vi "Complete_Controller_w_optics.vi"() -> ()   [LabVIEW 2014]
uses:
  <vilib>/LabVIEW Interface for Arduino/Type Defs/Arduino Resource.ctl
  <vilib>/LabVIEW Interface for Arduino/Type Defs/Board Type.ctl
  <vilib>/Instr/_visa.llb/VISA Configure Serial Port (Instr).vi
  <vilib>/Utility/file.llb/Write To Spreadsheet File (string).vi
  <vilib>/Utility/file.llb/Write To Spreadsheet File (DBL).vi
  <vilib>/Utility/file.llb/Read From Spreadsheet File (string).vi
  <vilib>/DAQmx/write.llb/DAQmx Write (Digital Bool 1Line 1Point).vi
  <vilib>/DAQmx/write.llb/DAQmx Write (Analog 1D DBL NChan 1Samp).vi
  <vilib>/DAQmx/read.llb/DAQmx Read (Analog 1D DBL NChan 1Samp).vi
  Environmental Chamber LabVIEW and Instruments/Drivers and Software/keithley_6430/Keithley 6430/Public/Data/Read (Single Point).vi
  Environmental Chamber LabVIEW and Instruments/Drivers and Software/LabVIEW 8.2 Drivers/keithley_24xx/Keithley 24XX/Public/Data/Read (Single Point).vi
  Environmental Chamber LabVIEW and Instruments/Drivers and Software/keithley_24xx/Keithley 24XX/Keithley 24XX.lvlib
  Environmental Chamber LabVIEW and Instruments/Drivers and Software/keithley_6430/Keithley 6430/Keithley 6430.lvlib
  <vilib>/LabVIEW Interface for Arduino/LabVIEW Interface for Arduino.lvlib
panel:
  in  "Integration Time (ms)":i32=80 caption="Inter scan delay ms"
  in  "Optical Smoothing Level":i32 min=0 max=4 step=1
  in  "Number of Scans to Average":i32=1 min=1 max=10000 step=1
  in  "Digitizer Clock Rate Setting":i32=3 min=1 max=3
  out "Critical Error":bool
  in  "Save spectra file path":path=path "C:/Users/User/Desktop/Chamber Data/perovskites/2015-08-04 spectra"
  in  "Aquire spectra":bool
  in  "Seconds between  spectra":dbl caption="Time Target (s)"
  out "Spectrum":cluster{"Wavelengths":dbl[], "buffer out":sgl[]}(graph)
  out "output param":i32
  out "Sequence time left (hrs)":dbl caption="min"
  out "Sequence Preview":cluster{dbl[], dbl[]}[](graph)
  out "Pressure Control 3":bool caption="Pressure Control"
  in  "valve % open":dbl=100.0 min=0.0 max=100.0 step=5.0
  in  "Vapor\nflow\n(sccm)":sgl(slide) min=0 max=100 step=1 scale=0.0..200.0
  out "Actual":dbl
  out "Boolean 3":bool
  out "Actual":dbl
  out "Boolean":bool
  in  "Gas\nflow\n(sccm)":sgl(slide) min=0 max=100 step=1 scale=0.0..200.0
  in  "Desired pressure":dbl min=0.0 max=760.0 step=5.0
  out "Valve position (%)":dbl
  in  "Pressure Control":enum32{"Set % open ", " Set pressure  (Torr)"}(radio)
  out "Pressure Control 2":bool caption="Pressure Control"
  out "Keithley 6430":bool
  out "J-Kem":bool caption="J-Kem Temp"
  out "J-Kem Temp (C)":cluster{dbl}(graph)
  out "Keithley 2420":bool caption="Keithley 2430"
  out "Pressure Control":bool
  out "SRS QCM":bool
  out "MHz":dbl format="%.6f"
  out "Ohm":dbl format="%.4e"
  out "Waveform Chart 7":cluster{dbl, "Resistance out":dbl}(graph)
  out "Chamber Pressure (Torr)":cluster{"f":dbl}(graph)
  in  "Start recording after":dbl caption="min"
  in  "Auto stop after":bool
  in  "hrs":dbl=1000.0 min=0.0
  out "Start Time":string
  out "Elapsed (min)":dbl caption="Elapsed Time (s)"
  in  "Delay between data points (s)":dbl caption="sec" min=0.0 max=30.0 format="%#_13g"
  in  "Turbo pump auto on":bool
  in  "stop":bool
  in  "Experiment Notes":string
  in  "Clear all charts":bool
  out "Save data file path":path
  out "Waveform Chart 2":cluster{"f":dbl, "f":dbl}(graph)
  out "Keithley 2420 (Ohm)":cluster{"Resistance":sgl}(graph)
  out "Keithley 6430 (Ohm)":cluster{"Measurement":dbl}(graph)
  in  "Tab Control":T1(tab)
  out "run sequence table":string[][](table) caption="Sequence to run"
  in  "Run Sequence":bool
  out "Current step":i32
  out "Step time remaining (min)":dbl caption="min" format="%#_1g"
  in  "Import sequence file":path
  in  "Use excel file\nfor sequence?":bool
  in  "Pressure Mode":T2(radio)
  in  "User-defined\nsequence":string[][](table) caption="Create sequence"
  in  "Partial pressure of solvent (%)":dbl=100.0 min=0.0 max=100.0 step=5.0
  out "Arduino":bool
  out "temp\n(C)":string
  out "gas\nsensor":string
  out "Arduino humidity (%)":cluster{dbl}(graph)
  out "QCM mass deposited (g)":cluster{dbl}(graph)
  in  "rapidox O2 Sensor":bool
  in  "setnag O2 Pump":bool
  in  "Baud Rate 2":i32(ring)=2 items=["2400", "4800", "9600", "19200", "38400", "57600", "115200"]
  in  "Com Port":i32(ring) items=["Com 1", "Com 2", "Com 3", "Com 4", "Com 5", "Com 6", "COM 7", "COM 8", "COM 9", "COM 10", "COM 11", "COM 12", "com 13", "COM 14"]
  in  "Com Port 2":i32(ring) items=["Com 1", "Com 2", "Com 3", "Com 4", "Com 5", "Com 6", "COM 7", "COM 8", "COM 9", "COM 10", "COM 11", "COM 12", "com 13", "COM 14"]
  out "Torr":dbl
  out "%":dbl
  out "atm":dbl
  out "Waveform Chart":cluster{dbl}(graph)
  out "O2 Concentration (PPM)":dbl
  out "Waveform Chart 6":cluster{dbl}(graph)
  # "Currently Unused"
  # "QCM"
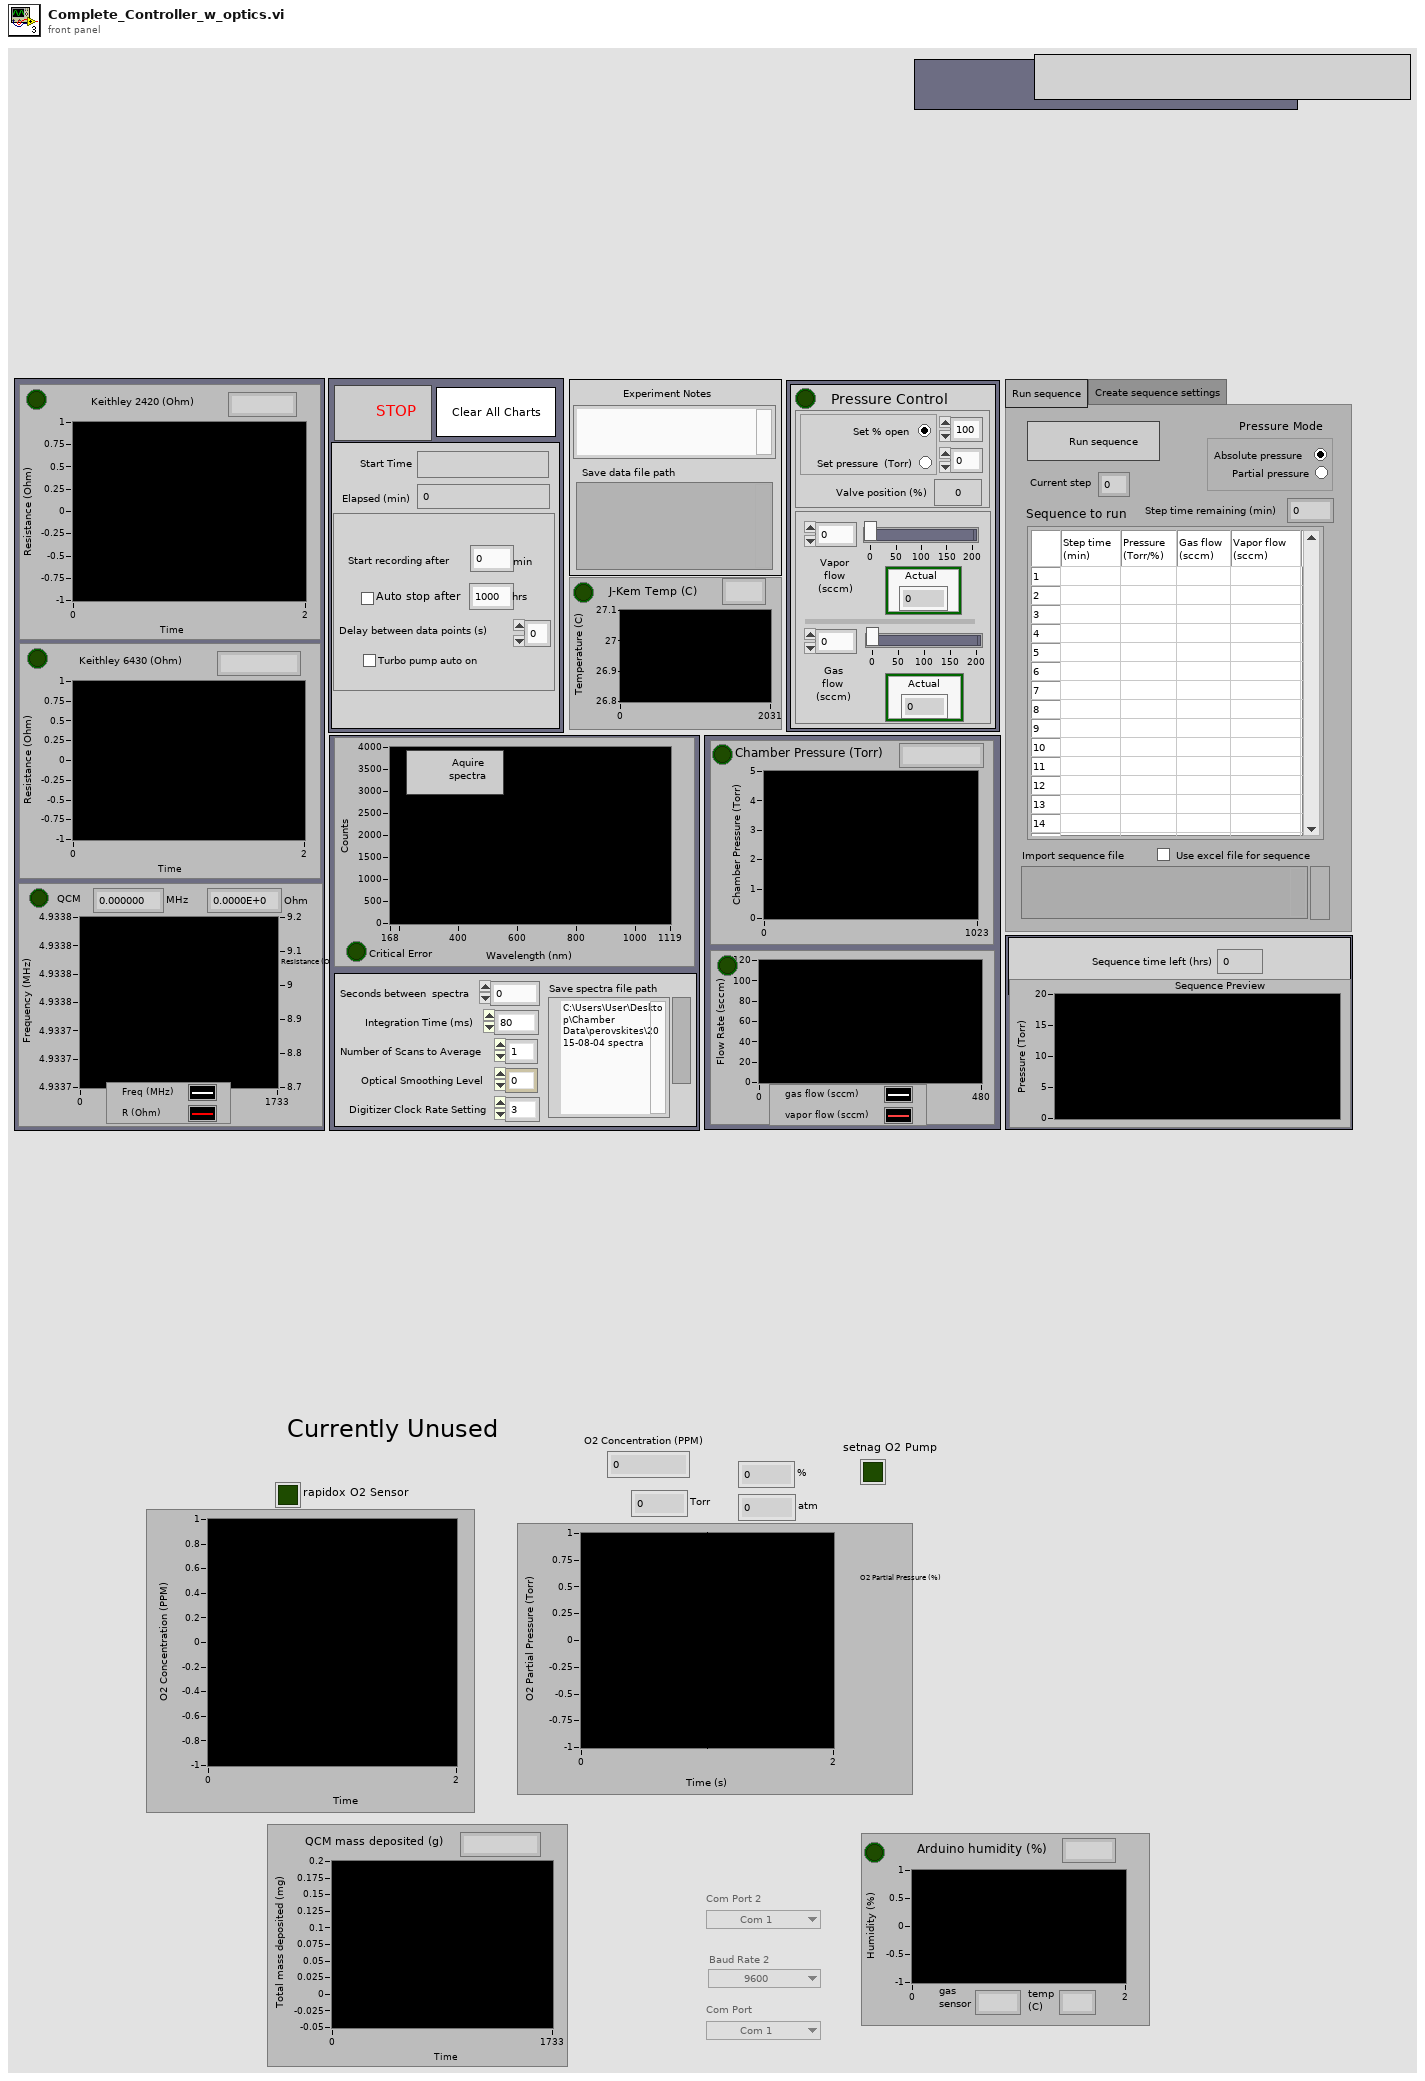
[diagram p1: front panel]
types:
  T1 = enum32{"Run sequence", "Create sequence settings"}
  T2 = enum32{"Absolute pressure ", " Partial pressure"}
  T3 = enum16{"open", "open or create", "create or replace", "create", "open (read only)"}
  T4 = enum16{"no parity", "odd parity", "even parity", "mark parity", "space parity"}
  T5 = cluster{bool, "VISA resource name":refnum<visa-resource-name>, "error out":errorcluster}
  T6 = cluster{bool, "VISA resource name out":refnum<visa-resource-name>, "error out":errorcluster}
  T7 = cluster{"task out":refnum<k21>, "error out":errorcluster, "task out":refnum<k21>, "error out":errorcluster, "task out":refnum<k21>, "error out":errorcluster, "VISA resource name":refnum<visa-resource-name>, "error out":errorcluster}
  T8 = cluster{"task out":refnum<k21>, "error out":errorcluster, "task out":refnum<k21>, "error out":errorcluster, "task out":refnum<k21>, "error out":errorcluster, "VISA resource name out":refnum<visa-resource-name>, "error out":errorcluster}
  T9 = cluster{"Coefficients":ext[], "Wavelengths":dbl[]}[]
  T10 = cluster{"Integration Time (ms)":i32, "Number of Scans to Average":i32, "Optical Smoothing Level":i32, "Digitizer Clock Rate Setting":i32, "Temp  Compensation ":bool}[]
  T11 = cluster{"Integration Time (ms)":i32, "Number of Scans to Average":i32, "Optical Smoothing Level":i32, "Digitizer Clock Rate Setting":i32, "Temp  Compensation ":bool}
  T12 = cluster{"Coefficients":ext[], "Wavelengths":dbl[]}
  T13 = cluster{bool, "VISA out":refnum<visa-resource-name>, "error out":errorcluster}
  T14 = cluster{"Boolean":bool, "VISA resource name out":refnum<visa-resource-name>, "error out":errorcluster}
  T15 = typedef "LabVIEW Interface for Arduino.lvlib/Arduino Resource.ctl" = cluster{"VISA resource":refnum<visa-resource-name>, "Board Type":T16, "Connection Type":enum8{"USB / Serial"}, "Bytes Per Packet (15)":u8}
  T16 = typedef "LabVIEW Interface for Arduino.lvlib/Board Type.ctl" = enum16{"Uno", "Dimuelanove w/Atmega 328", "Mega 2560"}
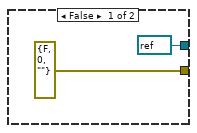
[diagram p3: hidden frame]
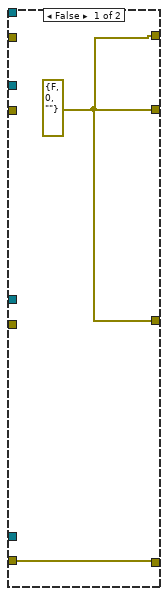
[diagram p4: hidden frame]
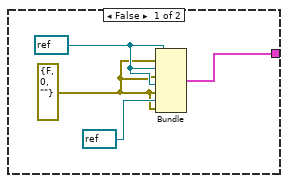
[diagram p5: hidden frame]
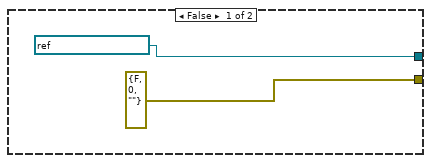
[diagram p7: hidden frame]
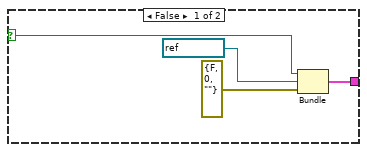
[diagram p8: hidden frame]
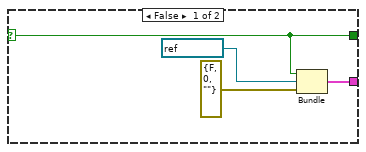
[diagram p10: hidden frame]
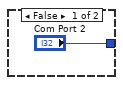
[diagram p11: hidden frame]
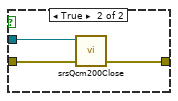
[diagram p12: hidden frame]
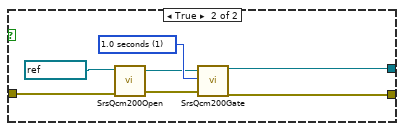
[diagram p13: hidden frame]
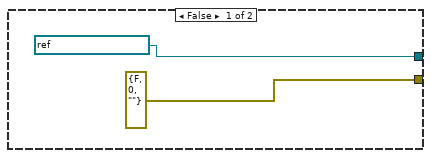
[diagram p15: hidden frame]
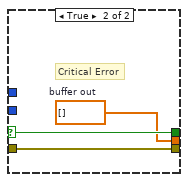
[diagram p17: hidden frame]
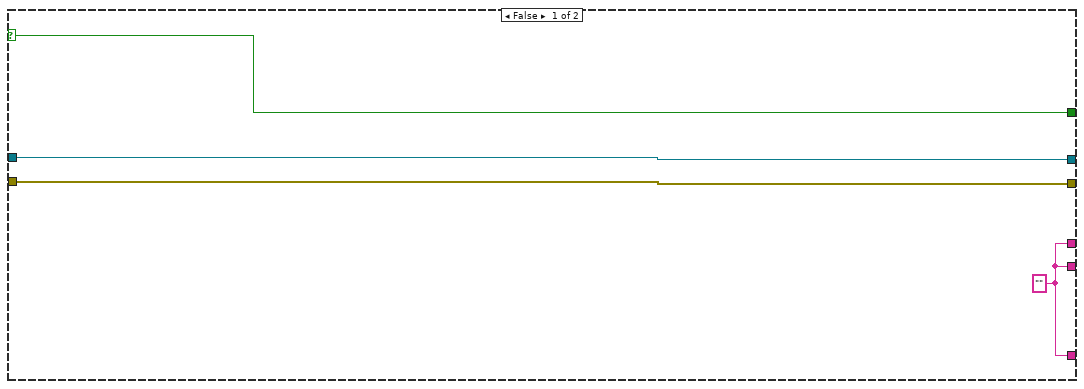
[diagram p18: hidden frame]
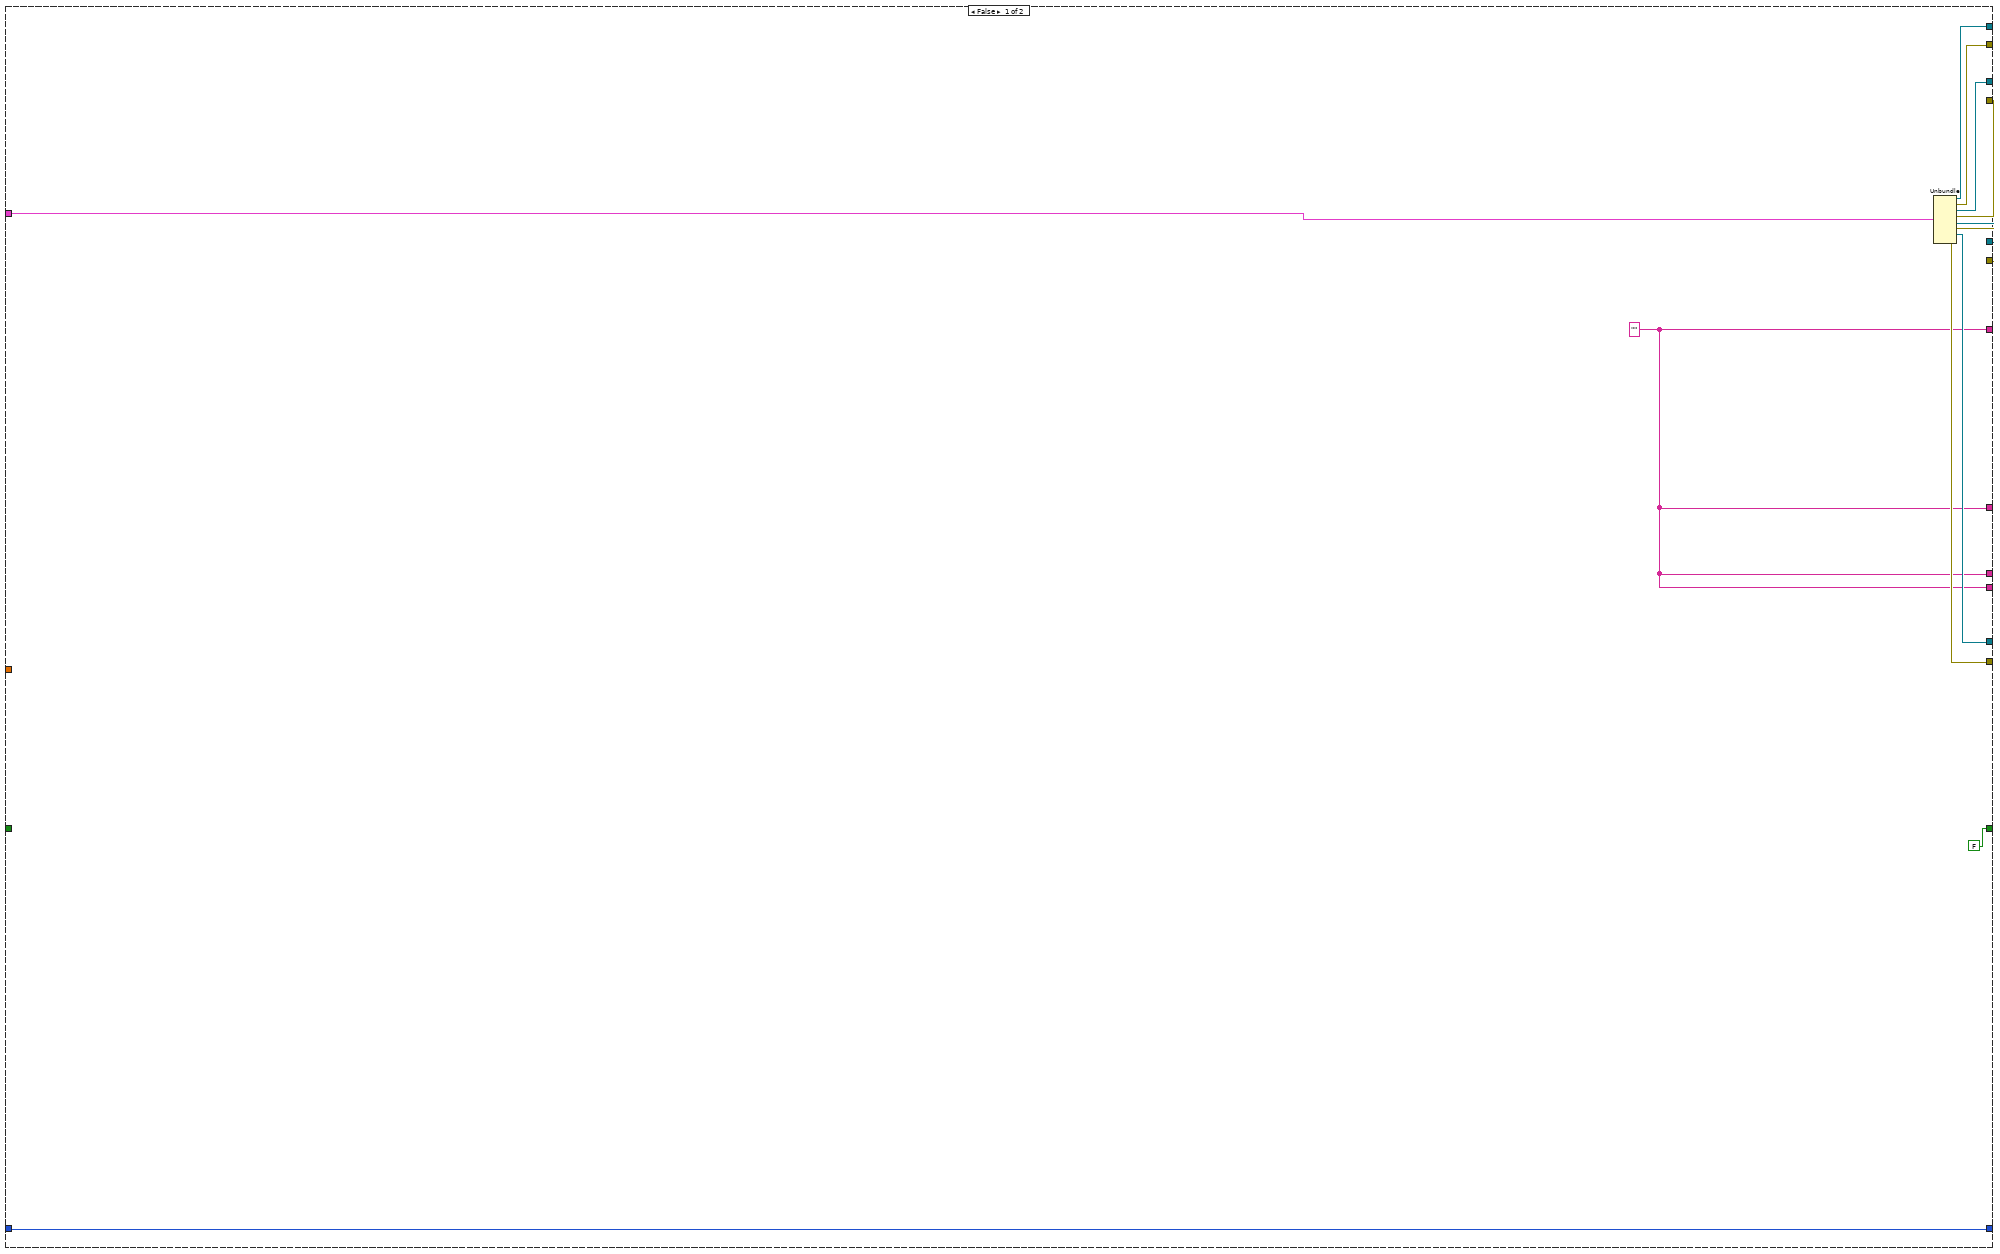
[diagram p19: hidden frame]
diagram:
  w29 = 0  # 1st step
  n1 = call "setup.vi"() -> ("Save file path 2"=w1:path, "begin recording"=w16:dbl, "error IO"=w4:errorcluster, "stop after"=w18:dbl, "Auto Stop 2"=w19:bool, "delay 5"=w17:dbl, "SRS QCM 2"=w15:bool, "Keithley 6431"=w11:bool, "Keithley 2421"=w14:bool, "J-KEM2"=w13:bool, "Arduino2"=w12:bool, "Pressure control 2"=w10:bool)  [unwired: 8 in]
  "SRS QCM" <- w15
  "Arduino" <- w12
  "Pressure Control" <- w10
  "Keithley 2420" <- w14
  "J-Kem" <- w13
  "Keithley 6430" <- w11
  "Pressure Control 2" <- w10
  "Pressure Control 3" <- w10
  n2 = local write "Auto stop after"(w19) -> ()
  n3 = local write "hrs"(w18) -> ()
  n4 = local write "Delay between data points (s)"(w17) -> ()
  n5 = local write "Start recording after"(w16) -> ()
  n6 = case shown="True" w14 {
    tunnel: [refnum<visa-resource-name> "GPIB1::24::INSTR" ("VISA resource name") w108] -> w96
    tunnel: [errorcluster {"status"=FALSE, "code"=0, "source"=""} ("error out") w103] -> w95
    frame False {
    }
    frame True {
      w110 = u16 0 items=["Voltage", "Current"] ("Source Mode  (0: Voltage)")
      w115 = u16 2 items=["Volts", "Current", "Resistance"] ("Function (0: Volts)")
      n7 = call "Initialize.vi"("VISA resource name"=refnum<visa-resource-name> "GPIB1::24::INSTR") -> ("error out"=w104:errorcluster, "VISA resource name out"=w107:refnum<visa-resource-name>)  [unwired: 9 in]
      n8 = call "Enable Remote Sensing.vi"("error in (no error)"=w104, "Enable Remote Sensing (T: Enable)"=FALSE ("4-wire?"), "VISA resource name"=w107) -> ("error out"=w105:errorcluster, "VISA resource name out"=w106:refnum<visa-resource-name>)  [unwired: 7 in]
      n9 = call "Configure Measurement.vi"("error in (no error)"=w105, "Function (0: Volts)"=w115, "VISA resource name"=w106) -> ("error out"=w114:errorcluster, "VISA resource name out"=w113:refnum<visa-resource-name>)  [unwired: 7 in]
      n10 = call "Configure Output.vi"("Source Mode  (0: Voltage)"=w110, "error in (no error)"=w114, "Output Level (0)"=0.1 ("Applied Voltage (V)"), "VISA resource name"=w113) -> ("error out"=w112:errorcluster, "VISA resource name out"=w111:refnum<visa-resource-name>)  [unwired: 6 in]
      n11 = call "Enable Output.vi"("error in (no error)"=w112, "VISA resource name"=w111) -> ("error out"=w103:errorcluster, "VISA resource name out"=w108:refnum<visa-resource-name>)  [unwired: 8 in]
    }
  }
  n12 = case shown="True" w11 {
    tunnel: [refnum<visa-resource-name> "GPIB0::29::INSTR" ("VISA resource name") w125] -> w53
    tunnel: [errorcluster {"status"=FALSE, "code"=0, "source"=""} ("error out") w126] -> w52
    frame False {
    }
    frame True {
      (unwired) 15000.0 ("Resistance Range [Ohms]")
      w121 = u16 0 items=["On", "Off", "Once"] ("Autozero  (0: On)")
      w129 = TRUE  # Output (F:Off)
      n13 = call "Initialize.vi"("VISA resource name"=refnum<visa-resource-name> "GPIB0::29::INSTR") -> ("error out"=w122:errorcluster, "VISA resource name out"=w123:refnum<visa-resource-name>)  [unwired: 4 in, 5 out]
      n14 = call "Configure Autozero.vi"("error in (no error)"=w122, "Autozero  (0: On)"=w121, "VISA resource name"=w123) -> ("error out"=w119:errorcluster, "VISA resource name out"=w120:refnum<visa-resource-name>)  [unwired: 7 in]
      n15 = call "Configure MeasureOhms.vi"("error in (no error)"=w119, "Auto Range (T:Enable)"=TRUE, "VISA resource name"=w120) -> ("error out"=w130:errorcluster, "VISA resource name out"=w128:refnum<visa-resource-name>)  [unwired: 3 in, 4 out]
      n16 = call "Enable Output.vi"("error in (no error)"=w130, "Enable Output (F:Off)"=w129, "VISA resource name"=w128) -> ("error out"=w126:errorcluster, "VISA resource name out"=w125:refnum<visa-resource-name>)  [unwired: 7 out]
    }
  }
  n17 = property on="Turbo pump auto on" class="Bool (strict)"(error in=w4, "Value"=TRUE ("Turbo\npump")) -> (error out=w3:errorcluster)  [unwired: 1 in, 1 out]
  n18 = case shown="True" "setnag O2 Pump" {
    tunnel: ["Com Port 2" w132] -> w92
    frame False {
    }
    frame True {
      n19 = flat-sequence {
        tunnel: ["Com Port"] -> w135
        tunnel: [w137] -> w134
        tunnel: ["Com Port"] -> w133
        tunnel: w135 -> [w143]
        tunnel: w134 -> [w142]
        tunnel: w133 -> [w144]
        tunnel: [w144] -> w132
        frame #0 {
          n20 = property on="Baud Rate 2" class="Ring (strict)"() -> ("Strings []"=w139:string[])  [unwired: 2 in, 2 out]
          n21 = Index Array(array=w139, index="Baud Rate 2") -> (element=w140:string)
          n22 = Decimal String To Number(string=w140) -> (number=w138:i32)  [unwired: 2 in, 1 out]
          n23 = To Unsigned Long Integer(number=w138) -> (unsigned 32bit integer=w137:u32)
        }
        frame #1 {
          n24 = call <vilib>:"Serial Port Init.vi"("parity"=T4."no parity", "buffer size"=u16 65535, "stop bits"=enum16{"1 bit", "1.5 bits", "2 bits"}."1 bit", "data bits"=u16 8, "baud rate"=w142, "port number"=w143) -> ()  [unwired: 1 in, 1 out]
        }
      }
    }
  }
  n25 = property on="Run Sequence" class="Bool (strict)"(error in=w3, "Value"=FALSE ("Run Sequence")) -> (error out=w8:errorcluster)  [unwired: 1 in, 1 out]
  n26 = case shown="True" "rapidox O2 Sensor" {
    selector: "rapidox O2 Sensor" -> [w149 w154]
    tunnel: [w150 w155] -> w63
    frame False {
      n27 = Bundle(w149, "VISA resource name"=refnum<visa-resource-name> "COM7", "error out"=errorcluster {"status"=FALSE, "code"=0, "source"=""}) -> (w150:T5)  [unwired: 1 in]
    }
    frame True {
      n28 = call-poly "VISA Configure Serial Port"("VISA resource name"=refnum<visa-resource-name> "COM7") -> ("VISA resource name out"=w156:refnum<visa-resource-name>, "error out"=w153:errorcluster)  [unwired: 13 in]
      n29 = Bundle(w154, "VISA resource name out"=w156, "error out"=w153) -> (w155:T6)  [unwired: 1 in]
    }
  }
  n30 = case shown="False" w15 {
    tunnel: [refnum<visa-resource-name> "COM6" ("VISA in") w162] -> w94
    tunnel: [w158 w161] -> w93
    tunnel: w8 -> [w158 w160]
    frame False {
    }
    frame True {
      w166 = u16 1 items=["0.1 seconds", "1.0 seconds", "10.0 seconds"] ("Gate in")
      n31 = call "SrsQcm200Open.vi"("error in"=w160, "VISA in"=refnum<visa-resource-name> "COM6") -> ("error out"=w163:errorcluster, "VISA out"=w164:refnum<visa-resource-name>)  [unwired: 3 in]
      n32 = call "SrsQcm200Gate.vi"("VISA in"=w164, "Gate in"=w166, "error in (no error)"=w163) -> ("VISA out"=w162:refnum<visa-resource-name>, "error out"=w161:errorcluster)  [unwired: 14 in, 1 out]
    }
  }
  n33 = case shown="True" w10 {
    tunnel: [w167 w174] -> w34
    frame False {
      w169 = refnum<k21> refnum ("task out")
      w168 = errorcluster {"status"=FALSE, "code"=0, "source"=""} ("error out")
      n34 = Bundle("task out"=w169, "error out"=w168, "task out"=w169, "error out"=w168, "task out"=w169, "error out"=w168, "VISA resource name"=refnum<visa-resource-name> refnum, "error out"=w168) -> (w167:T7)  [unwired: 1 in]
    }
    frame True {
      # "Turbo Pump Control"
      # "DAQ Gas/Vapor Flow Readings"
      # "DAQ Pressure Readings"
      # "Butterfly Valve"
      n35 = call-poly "VISA Configure Serial Port"("VISA resource name"=refnum<visa-resource-name> "COM5") -> ("VISA resource name out"=w175:refnum<visa-resource-name>, "error out"=w171:errorcluster)  [unwired: 13 in]
      n36 = call <vilib>:"DAQmx Start Task.vi"("task/channels in"=refnum<k21> "AllDaqReadings") -> ("task out"=w177:refnum<k21>, "error out"=w176:errorcluster)  [unwired: 13 in]
      n37 = call <vilib>:"DAQmx Start Task.vi"("task/channels in"=refnum<k21> "TurboON") -> ("task out"=w181:refnum<k21>, "error out"=w180:errorcluster)  [unwired: 13 in]
      n38 = call <vilib>:"DAQmx Start Task.vi"("task/channels in"=refnum<k21> "Setflow") -> ("task out"=w179:refnum<k21>, "error out"=w178:errorcluster)  [unwired: 13 in]
      n39 = property on="Run Sequence" class="Bool (strict)"(error in=w171, "Value"=FALSE ("Run Sequence")) -> (error out=w173:errorcluster)  [unwired: 1 in, 1 out]
      n40 = Bundle("task out"=w181, "error out"=w180, "task out"=w179, "error out"=w178, "task out"=w177, "error out"=w176, "VISA resource name out"=w175, "error out"=w173) -> (w174:T8)  [unwired: 1 in]
    }
  }
  n41 = case shown="True" w13 {
    selector: w13 -> [w186 w191]
    tunnel: [w187 w192] -> w81
    tunnel: [w186 w191] -> w75
    frame False {
      n42 = Bundle(w186, "VISA resource name"=refnum<visa-resource-name> "COM3", "error out"=errorcluster {"status"=FALSE, "code"=0, "source"=""}) -> (w187:T5)  [unwired: 1 in]
    }
    frame True {
      n43 = call-poly "VISA Configure Serial Port"("VISA resource name"=refnum<visa-resource-name> "COM3") -> ("VISA resource name out"=w193:refnum<visa-resource-name>, "error out"=w190:errorcluster)  [unwired: 13 in]
      n44 = Bundle(w191, "VISA resource name out"=w193, "error out"=w190) -> (w192:T6)  [unwired: 1 in]
    }
  }
  n45 = Get Date/Time In Seconds() -> (seconds since 1Jan1904=w99:timestamp)
  n46 = case "Arduino" shown="True" w12 {
    tunnel: [refnum<visa-resource-name> refnum ("VISA resource name out") w200] -> w28
    tunnel: [errorcluster {"status"=FALSE, "code"=0, "source"=""} ("error out") w197] -> w27
    frame False {
    }
    frame True {
      n47 = call <vilib>:"Init.vi"() -> ()  [unwired: 18 in, 2 out]
      n48 = call-poly "VISA Configure Serial Port"("VISA resource name"=refnum<visa-resource-name> "COM12", "baud rate (9600)"=u32 9600) -> ("VISA resource name out"=w200:refnum<visa-resource-name>, "error out"=w197:errorcluster)  [unwired: 12 in]
    }
  }
  n49 = Format Date/Time String(seconds (now)=w99) -> (date/time string=→"Start Time":string)  [unwired: 2 in]
  n50 = call "OpenCreateReplace File.vi"("function (open:0)"=T3."create or replace", "file path"=w1) -> ("new file path"=w20:path)  [unwired: 6 in, 3 out]
  "Save data file path" <- w20
  n51 = while {
    shift-right: [w296] -> _
    shift-left: _ -> [w295]
    tunnel: [w225] -> w97 mode=indexing if=w224
    tunnel: w14 -> [w264]
    tunnel: w96 -> [w293]
    tunnel: w95 -> [w292]
    tunnel: w94 -> [w291]
    tunnel: w93 -> [w290]
    tunnel: w15 -> [w288]
    tunnel: "setnag O2 Pump" -> [w281]
    tunnel: w92 -> [w287]
    tunnel: [w283] -> w89
    tunnel: [w282] -> w85
    tunnel: w81 -> [w280]
    tunnel: [w279] -> w80
    tunnel: w75 -> [w277]
    tunnel: w63 -> [w273]
    tunnel: [w268] -> w61
    tunnel: [w263] -> w60
    tunnel: w20 -> [w263]
    shift-right: [w246] -> _
    shift-left: _ -> [w248]
    tunnel: w53 -> [w260]
    tunnel: w52 -> [w259]
    tunnel: [w258] -> w51
    tunnel: w11 -> [w257]
    tunnel: w10 -> [w238]
    tunnel: [w254] -> w47
    tunnel: [w253] -> w44
    tunnel: [w252] -> w46
    tunnel: [w251] -> w45
    tunnel: [w238] -> w43
    tunnel: [w250] -> w38
    tunnel: w34 -> [w242]
    tunnel: [w241] -> w32
    tunnel: [w240] -> w31
    tunnel: [w239] -> w30
    shift-right: [w237] -> _
    shift-left: w29 -> [w236]
    tunnel: w12 -> [w221]
    tunnel: w28 -> [w231]
    tunnel: w27 -> [w230]
    tunnel: [w229] -> w26
    tunnel: [w228] -> w25
    tunnel: [w227] -> w24
    shift-right: [w212] -> _
    shift-left: TRUE -> [w213]
    i -> [w210]
    stop <- w276 stop-if-true
    n52 = call "Elapsed Time"() -> ("Present (s)"=w235:dbl, "Elapsed Time (s)"=w275:dbl)  [unwired: 12 in, 6 out]
    n53 = call "Elapsed Time5"("Time Target (s)"="Seconds between  spectra", "Auto Reset"=TRUE) -> ("Time has Elapsed"=w204:bool)  [unwired: 10 in, 7 out]
    n54 = Divide(x=w275, y=60.0) -> (x/y=w215:dbl)
    "Elapsed (min)" <- w215
    n55 = And(x=w204, y="Aquire spectra") -> (x .and. y?=w202:bool)
    n56 = Greater Or Equal?(x=w215, y="Start recording after") -> (x >= y?=w224:bool)
    n57 = Multiply(x="hrs", y=60.0) -> (x*y=w207:dbl)
    n58 = case "Vacuum / Pressure / Sequence" shown="True" w238 {
      tunnel: [w395 w503] -> w253
      tunnel: [w396 w502] -> w251
      tunnel: [w398 w483] -> w254
      tunnel: [w397 w484] -> w252
      tunnel: [w396 w474] -> w250
      tunnel: [w391 w464] -> w245
      tunnel: [w391 w463] -> w244
      tunnel: [w391 w461] -> w243
      tunnel: w242 -> [w401 w459]
      tunnel: [w400 w450] -> w241
      tunnel: [w399 w449] -> w240
      tunnel: [w394 w448] -> w239
      tunnel: w236 -> [w393 w433]
      tunnel: [w393 w445] -> w237
      tunnel: w235 -> [_ w444]
      tunnel: w213 -> [_ w424]
      tunnel: [FALSE ("new element/subarray") w419] -> w212
      tunnel: [w391 w418] -> w211
      frame False {
        w391 = ""
        n59 = Unbundle(w401) -> ("task out"=w400:refnum<k21>, "error out"=w399:errorcluster, "task out"=w398:refnum<k21>, "error out"=w397:errorcluster, "task out"=w395:refnum<k21>, "error out"=w396:errorcluster, "VISA resource name out"=w394:refnum<visa-resource-name>)  [unwired: 1 out]
      }
      frame True {
        # "system info"
        # "DAQ Pressure, Gas/Vapor Flows, & Butterfly Valve Control"
        n60 = case shown="True" "Use excel file\nfor sequence?" {
          tunnel: ["User-defined\nsequence" w510] -> w410
          frame False {
          }
          frame True {
            n61 = call-poly <vilib>:"Read From Spreadsheet File.vi"("file path (dialog if empty)"="Import sequence file") -> ("all rows"=w512:string[][])  [unwired: 6 in, 4 out]
            n62 = for {
              tunnel: w512 -> [w514] mode=indexing
              tunnel: [w513] -> w510 mode=indexing
              n63 = for {
                tunnel: w514 -> [w516] mode=indexing
                tunnel: [w515] -> w513 mode=indexing
                n64 = Format Into String(w516) -> (resulting string=w515:string)  [unwired: 3 in, 1 out]
              }
            }
          }
        }
        "run sequence table" <- w410
        n65 = case shown="\" Partial pressure\"" "Pressure Mode" {
          tunnel: [w505 w507] -> w402
          tunnel: "Desired pressure" -> [w505 w506]
          frame "Absolute pressure ", Default {
          }
          frame " Partial pressure" {
            n66 = Divide(x=w506, y="Partial pressure of solvent (%)") -> (x/y=w507:dbl)
          }
        }
        n67 = Unbundle(w459) -> ("task out"=w452:refnum<k21>, "error out"=w451:errorcluster, "task out"=w453:refnum<k21>, "error out"=w454:errorcluster, "task out"=w455:refnum<k21>, "error out"=w456:errorcluster, "VISA resource name out"=w457:refnum<visa-resource-name>, "error out"=w458:errorcluster)
        n68 = Wait (ms)(milliseconds to wait=u32 1000) -> ()  [unwired: 1 out]
        n69 = Fract/Exp String To Number(string=w410) -> (number=w423:dbl[][])  [unwired: 3 in, 1 out]
        n70 = call "plot_usr_seq.vi"("User-defined sequence"=w410) -> ("Sequence Preview"=→"Sequence Preview":cluster{dbl[], dbl[]}[])
        n71 = Index Array(array=w423, index (col)=0 ("disabled index (col)")) -> (element=w437:dbl[])  [unwired: 1 in]
        n72 = Index Array "time"(array=w423, index (row)=0 ("disabled index (col)")) -> (element=w422:dbl[])  [unwired: 1 in]
        n73 = Add Array Elements(numeric array=w437) -> (sum=w428:dbl)
        n74 = Array Size(array=w422) -> ()  [unwired: 1 out]
        n75 = call-poly <vilib>:"DAQmx Read.vi"("task/channels in"=w455, "error in"=w456) -> ("task out"=w503:refnum<k21>, "data"=w494:dbl[], "error out"=w502:errorcluster)  [unwired: 11 in]
        n76 = And(x="Run Sequence", y=w424) -> (x .and. y?=w425:bool)
        n77 = case "Sequence" shown="True" w425 {
          tunnel: w444 -> [_ w553]
          tunnel: [w539 w554] -> w445
          tunnel: w433 -> [w539 w541]
          tunnel: "Vapor\nflow\n(sccm)" -> [w538 _]
          tunnel: "Gas\nflow\n(sccm)" -> [w537 _]
          tunnel: [w538 w562] -> w441
          tunnel: [w537 w561] -> w440
          tunnel: [w536 w560] -> w429
          tunnel: w402 -> [w536 _]
          tunnel: w423 -> [_ w547]
          tunnel: "Pressure Control" -> [w535 _]
          tunnel: [w535 enum32{"Open Mode", "Pressure Mode"}."Pressure Mode" ("Pressure Control")] -> w434
          tunnel: [0.0 w550] -> w427
          frame False {
          }
          frame True {
            # "User Sequence"
            n78 = Array Size(array=w547) -> (size(s)=w570:i32[])
            n79 = Index Array "gas flow"(array=w547, index (row)=w541, index (col)=2 ("disabled index (col)")) -> (element=w561:dbl)
            n80 = Index Array "Pressure"(array=w547, index (row)=w541, index (col)=1 ("disabled index (col)")) -> (element=w560:dbl)
            n81 = Index Array "vapor flow"(array=w547, index (row)=w541, index (col)=3 ("disabled index (col)")) -> (element=w562:dbl)
            n82 = Index Array "array length"(array=w570) -> (element=w548:i32)  [unwired: 1 in]
            n83 = Index Array "time"(array=w547, index (row)=w541, index (col)=0) -> (element=w559:dbl)
            n84 = Greater Or Equal?(x=w548, y=w541) -> (x >= y?=w567:bool)
            n85 = Multiply(x=w559, y=60.0) -> (x*y=w546:dbl)
            n86 = call "Elapsed Time3"("Time Target (s)"=w546, "Auto Reset"=TRUE, "Set Start Time (s)"=w553) -> ("Elapsed Time (s)"=w545:dbl, "Time has Elapsed"=w566:bool)  [unwired: 9 in, 6 out]
            n87 = Increment(x=w541) -> (x+1=→"Current step":i32)
            n88 = Subtract(x=w546, y=w545) -> (x-y=w542:dbl)
            n89 = And(x=w566, y=w567) -> (x .and. y?=w556:bool)
            n90 = call "Elapsed Time4"("Reset"=FALSE, "Set Start Time (s)"=w553) -> ("Elapsed Time (s)"=w551:dbl)  [unwired: 10 in, 7 out]
            n91 = Increment(x=w541) -> (x+1=w555:i32)
            n92 = Divide(x=w542, y=60.0) -> (x/y=→"Step time remaining (min)":dbl)
            n93 = Select(t=w555, s=w556, f=w541) -> (s? t:f=w554:i32)
            n94 = Divide(x=w551, y=60.0) -> (x/y=w550:dbl)
          }
        }
        n95 = Index Array "vapor flow"(array=w494, index=4) -> (element=w490:dbl)
        n96 = Index Array "vacuum presure"(array=w494, index=0) -> ()  [unwired: 1 out]
        n97 = Index Array "high pressure"(array=w494, index=1) -> (element=w497:dbl)
        n98 = Index Array "low pressure"(array=w494, index=2) -> (element=w468:dbl)
        n99 = Index Array "gas flow"(array=w494, index=3) -> (element=w492:dbl)
        n100 = Greater Or Equal To 0?(x=w468) -> (x >= 0?=w469:bool)
        n101 = Multiply(x=40.0, y=w490) -> (x*y=w481:dbl)
        n102 = Multiply(x=40.0, y=w492) -> (x*y=w478:dbl)
        n103 = Greater Or Equal?(x=w478, y=1.0) -> (x >= y?=w477:bool)
        n104 = Select(t=w468, s=w469, f=0.0) -> (s? t:f=w467:dbl)
        n105 = Greater Or Equal?(x=w481, y=1.0) -> (x >= y?=w480:bool)
        n106 = Multiply(x=100.0, y=w497) -> (x*y=w485:dbl)
        n107 = Select(t=w478, s=w477, f=0.0) -> (s? t:f=w412:dbl)
        "Actual" <- w412
        n108 = Select(t=w481, s=w480, f=0.0) -> (s? t:f=w411:dbl)
        "Actual" <- w411
        n109 = Greater?(x=w467, y=10.0) -> (0:w473:bool)
        n110 = Greater Or Equal To 0?(x=w485) -> (x >= 0?=w487:bool)
        n111 = Select(t=w485, s=w487, f=0.0) -> (s? t:f=w472:dbl)
        n112 = Bundle("f"=w412, "f"=w411) -> (→"Waveform Chart 2":cluster{"f":dbl, "f":dbl})  [unwired: 1 in]
        n113 = Greater Than 0?(x=w412) -> (x > 0?=→"Boolean 3":bool)
        n114 = Select(t=w472, s=w473, f=w467) -> (s? t:f=w414:dbl)
        n115 = Greater Than 0?(x=w411) -> (x > 0?=→"Boolean":bool)
        n116 = Greater?(x=0.05, y=w414) -> (0:w438:bool)
        n117 = Bundle("f"=w414) -> (→"Chamber Pressure (Torr)":cluster{"f":dbl})  [unwired: 1 in]
        n118 = And(x=w438, y="Turbo pump auto on") -> (x .and. y?=w446:bool)
        n119 = Number To Engineering String(4:w412) -> (0:w463:string)  [unwired: 3 in]
        n120 = Number To Engineering String(4:w414) -> (0:w464:string)  [unwired: 3 in]
        n121 = Number To Engineering String(4:w411) -> (0:w461:string)  [unwired: 3 in]
        n122 = Build Array(w441, w440) -> (w439:dbl[])
        n123 = Subtract(x=w428, y=w427) -> (x-y=w407:dbl)
        n124 = Equal To 0?(x=w412) -> (x = 0?=w416:bool)
        n125 = Equal To 0?(x=w411) -> (x = 0?=w417:bool)
        n126 = Divide(x=w407, y=60.0) -> (x/y=→"Sequence time left (hrs)":dbl)
        n127 = And(x=w416, y=w417) -> (x .and. y?=w415:bool)
        n128 = case shown="False" w415 {
          tunnel: w414 -> [w518 w528]
          tunnel: [w517 w527] -> w413
          tunnel: w412 -> [w526 _]
          tunnel: w411 -> [w524 _]
          frame False {
            # "Calculate humidity when gas/vapor are flowing"
            n129 = Add(x=w526, y=w524) -> (x+y=w525:dbl)
            n130 = Divide(x=w524, y=w525) -> (x/y=w519:dbl)
            n131 = Multiply(x=w518, y=w519) -> (x*y=w520:dbl)
            n132 = Divide(x=w520, y=23.8) -> (x/y=w522:dbl)
            n133 = Multiply(x=w522, y=100.0) -> (x*y=w517:dbl)
          }
          frame True {
            # "calculate humidity when no gas/vapor are flowing"
            n134 = Divide(x=w528, y=23.8) -> (x/y=w530:dbl)
            n135 = Multiply(x=w530, y=100.0) -> (x*y=w527:dbl)
          }
        }
        n136 = Less Or Equal To 0?(x=w407) -> (x <= 0?=w420:bool)
        n137 = case "reinitialize \"run sequence\" button  when sequence ends" shown="True" w420 {
          tunnel: [TRUE ("Run Sequence") w533] -> w419
          frame False {
          }
          frame True {
            w533 = FALSE ("Run Sequence")
            n138 = property on="Run Sequence" class="Bool (strict)"("Value"=w533) -> ()  [unwired: 2 in, 2 out]
          }
        }
        n139 = call "butterfly_valve_subvi.vi"("Desired pressure"=w429, "error in (no error)"=w458, "Pressure Control"=w434, 10:"valve % open", "VISA Refnum in"=w457) -> ("error out"=w474:errorcluster, "Valve position (%)"=→"Valve position (%)":dbl, "VISA Refnum out"=w448:refnum<visa-resource-name>)  [unwired: 4 in]
        n140 = call-poly <vilib>:"DAQmx Write.vi"("task/channels in"=w452, "data"=w446, "error in"=w451) -> ("task out"=w450:refnum<k21>, "error out"=w449:errorcluster)  [unwired: 10 in, 1 out]
        n141 = Number To Engineering String(4:w413) -> (0:w418:string)  [unwired: 3 in]
        n142 = Divide(x=w439, y=40.0 ("Waveform")) -> (x/y=w476:dbl[])
        n143 = call-poly <vilib>:"DAQmx Write.vi"("task/channels in"=w453, "data"=w476, "error in"=w454) -> ("task out"=w483:refnum<k21>, "error out"=w484:errorcluster)  [unwired: 10 in, 1 out]
      }
    }
    n144 = case shown="True" w202 {
      frame False {
      }
      frame True {
        w313 = 0 ("Spectral Channel")
        w315 = 1 ("Spectral Channel")
        w319 = FALSE ("Temp  Compensation")
        w327 = path "C:/program files/StellarNet/SpectraWiz"  # Location of SpectraWiz
        w337 = path "sw.ini"  # Name of SpectraWiz initialization file
        w329 = path "StellarNet init-read-close parameters.xml"  # Operating Parameters file
        w338 = path "StellarNet init-read-close coeffs.xml"  # Spectrometer Coefficients file
        # "StellarNet Spectrometer"
        # "Operation of the StellarNet spectrometers in LabVIEW\nis pretty simple.  See documentation in yellow boxes\non this diagram.  Essential steps are:\n\no  init the DLL\no  init (and count) the spectrometers connected\n\nFor each spectrometer you'll be working with:\n\no  manage the operating parameters (we have subVIs\n     which save/retrieve these from XML files so you\n     can always start with your previous parameters)\no  Take an initial scan and discard it\no  Scan away!"
        # "initialize the StellarNet .dll"
        # "To remember user and system settings, we store a few \nXML files.  If the files don't exist, they are created.\n\nRecent StellarNet LabVIEW applications all use the same\nXML file formats for storing user parameters, etc., but files\nfor each application are named uniquely to the \napplication."
        # "Find all connected spectrometers.  Retrieve parameters from stored files or EEPROM.  (Ask if all else fails)."
        # "selected spectrometer's\ncoeff's & wls"
        # "Multi-channel coeffs & wls"
        # "Multi-channel params"
        # "discard first scan"
        n145 = Build Path(base path=w327, name or relative path="swdll.dll") -> (appended path=w325:path)
        n146 = dll-call lib="C:/Program Files/StellarNet/SpectraWiz/swdll.dll" fn="SWDinit" label="init"(path in=w325) -> (error out=w326:errorcluster)  [unwired: 3 in, 1 out]
        n147 = call "StellarNet Initialize All Spectrometers, ext precision.vi"("Path of swdll.dll"=w325, "error in"=w326, "Spectrometer Coefficients file"=w338, "Location of SpectraWiz"=w327, "Name of SpectraWiz initialization file"=w337) -> ("error out"=w336:errorcluster, "Multi Channel Coeffs & WLs"=w334:T9, "Number of Channels"=w335:i32)  [unwired: 2 in, 2 out]
        n148 = call "StellarNet Initialize Operating Parameters.vi"("error in"=w336, "Spectrometer Coefficients file"=w329, "Location of SpectraWiz"=w327, "Number of Channels"=w335) -> ("error out"=w332:errorcluster, "Operating Parameters"=w330:T10)  [unwired: 6 in]
        n149 = Index Array(array=w330, index=w313) -> (element=w331:T11)
        n150 = Index Array(array=w334, index=w313) -> (element=w333:T12)
        n151 = Unbundle By Name(w333) -> ("Wavelengths"=w317:dbl[])  [unwired: 1 out]
        n152 = Bundle By Name(cluster=w331, "Integration Time (ms)"="Integration Time (ms)", "Optical Smoothing Level"="Optical Smoothing Level", "Number of Scans to Average"="Number of Scans to Average", "Digitizer Clock Rate Setting"="Digitizer Clock Rate Setting", "Temp  Compensation"=w319) -> (w322:T11)
        n153 = Replace Array Subset(array=w330, new element=w322, index=w313) -> ()  [unwired: 1 out]
        n154 = call "StellarNet Set Parameters.vi"("Temp  Compensation"=w319, "Digitizer Clock Rate Setting"="Digitizer Clock Rate Setting", "error in (no error)"=w332, "Optical Smoothing Level"="Optical Smoothing Level", "Number of Scans to Average"="Number of Scans to Average", "Integration Time (ms)"="Integration Time (ms)") -> ("error out"=w318:errorcluster)  [unwired: 5 in]
        n155 = call "StellarNet Scan.vi"("error in (no error)"=w318, "Integration Time (msec)"="Integration Time (ms)", "Spectral Channel"=w315) -> ("error out"=w343:errorcluster, "Critical Error"=w344:bool, "output param"=→"output param":i32)  [unwired: 5 in, 1 out]
        n156 = case shown="False" w344 {
          selector: w344 -> [_ w355]
          tunnel: w315 -> [w352 _]
          tunnel: [w351 w354] -> w328
          tunnel: [w349 w355] -> w341
          tunnel: w343 -> [w348 w353]
          tunnel: [w347 w353] -> w314
          tunnel: "Integration Time (ms)" -> [w346 _]
          frame False {
            n157 = call "StellarNet Scan.vi"("error in (no error)"=w348, "Integration Time (msec)"=w346, "Spectral Channel"=w352) -> ("error out"=w347:errorcluster, "buffer out"=w351:sgl[], "Critical Error"=w349:bool, "output param"=w350:i32)  [unwired: 5 in]
            n158 = local write "output param"(w350) -> ()
          }
          frame True {
            w354 = sgl[] []  # buffer out
            # "Critical Error"
          }
        }
        "Critical Error" <- w341
        n159 = Get Date/Time In Seconds() -> (seconds since 1Jan1904=w308:timestamp)
        n160 = Format Date/Time String(time format string (%c)="%Y-%m-%d %H_%M_%S", seconds (now)=w308) -> (date/time string=w303:string)  [unwired: 1 in]
        n161 = Split 1D Array(array=w328, index=2047) -> (first subarray=w316:sgl[])  [unwired: 1 out]
        n162 = Concatenate Strings(w303, ".txt") -> (w304:string)
        n163 = call <vilib>:"Simple Error Handler.vi"("error in (no error)"=w314) -> ()  [unwired: 4 in, 5 out]
        n164 = Build Array("wavelength (nm)", "intensity (a.u.)", w303) -> (w299:string[])
        n165 = Bundle("Wavelengths"=w317, w316) -> (→"Spectrum":cluster{"Wavelengths":dbl[], sgl[]})  [unwired: 1 in]
        n166 = Build Array(w317, w316) -> (w302:dbl[][])
        n167 = Build Path(base path="Save spectra file path", name or relative path=w304) -> (appended path=w306:path)
        n168 = Transpose 2D Array(2D array=w302) -> (transposed array=w301:dbl[][])
        n169 = call-poly <vilib>:"Write To Spreadsheet File.vi"("1D data"=w299, "file path (dialog if empty)"=w306) -> ("new file path (Not A Path if cancelled)"=w300:path)  [unwired: 6 in]
        n170 = call-poly <vilib>:"Write To Spreadsheet File.vi"("append to file? (new file:F)"=TRUE, "2D data"=w301, "file path (dialog if empty)"=w300) -> ()  [unwired: 5 in, 1 out]
      }
    }
    n171 = case "Clear all graphs" shown="True" "Clear all charts" {
      frame False {
      }
      frame True {
        w595 = cluster{dbl, "Resistance out":dbl}[] [] ("History Data")
        w594 = cluster{dbl}[] [] ("History Data")
        n172 = property on="Keithley 2420 (Ohm)" class="WFChart (strict)"("History Data"=w594) -> ()  [unwired: 2 in, 2 out]
        n173 = property on="J-Kem Temp (C)" class="WFChart (strict)"("History Data"=w594) -> ()  [unwired: 2 in, 2 out]
        n174 = property on="Keithley 6430 (Ohm)" class="WFChart (strict)"("History Data"=w594) -> ()  [unwired: 2 in, 2 out]
        n175 = property on="Waveform Chart 7" class="WFChart (strict)"("History Data"=w595) -> ()  [unwired: 2 in, 2 out]
        n176 = property on="Waveform Chart" class="WFChart (strict)"("History Data"=w594) -> ()  [unwired: 2 in, 2 out]
        n177 = property on="Waveform Chart 6" class="WFChart (strict)"("History Data"=w594) -> ()  [unwired: 2 in, 2 out]
        n178 = property on="QCM mass deposited (g)" class="WFChart (strict)"("History Data"=w594) -> ()  [unwired: 2 in, 2 out]
        n179 = property on="flow rates" class="WFChart (strict)"("History Data"=w595) -> ()  [unwired: 2 in, 2 out]
        n180 = property on="Chamber Pressure (Torr)" class="WFChart (strict)"("History Data"=w594) -> ()  [unwired: 2 in, 2 out]
        n181 = property on="Arduino humidity (%)" class="WFChart (strict)"("History Data"=w594) -> ()  [unwired: 2 in, 2 out]
      }
    }
    n182 = Number To Engineering String "elapsed time (min)"(4:w215) -> (0:w297:string)  [unwired: 3 in]
    n183 = Greater Or Equal?(x=w215, y=w207) -> (x >= y?=w218:bool)
    n184 = And(x=w218, y="Auto stop after") -> (x .and. y?=w216:bool)
    n185 = Or(x="stop", y=w216) -> (x .or. y?=w276:bool)
    n186 = Equal To 0?(x=w210) -> (x = 0?=w249:bool)
    n187 = Multiply(x=u32 1000, y="Delay between data points (s)") -> (x*y=w267:dbl)
    n188 = case "Setnag O2 Pump" shown="True" w281 {
      tunnel: [w666 w670] -> w296
      tunnel: w295 -> [w666 w671]
      tunnel: w267 -> [_ w667]
      tunnel: w287 -> [_ w669]
      tunnel: ["" w668] -> w286
      frame False {
      }
      frame True {
        # "SetNag O2 Gauge"
        n189 = flat-sequence {
          tunnel: [w680] -> w677
          tunnel: w667 -> [w682]
          tunnel: w669 -> [w680]
          tunnel: w677 -> [w683]
          tunnel: w667 -> [w690]
          tunnel: [w686] -> w670
          frame #0 {
            n190 = Wait (ms)(milliseconds to wait=w682) -> ()  [unwired: 1 out]
            n191 = call <vilib>:"Serial Port Write.vi"("string to write"="_OXY\r" ("O2 partial press"), "port number"=w680) -> ()  [unwired: 1 out]
          }
          frame #1 {
            # "O2 partial pressure"
            n192 = call <vilib>:"Bytes At Serial Port.vi"() -> ("byte count"=w691:u32)  [unwired: 1 in, 1 out]
            n193 = Wait (ms)(milliseconds to wait=w690) -> ()  [unwired: 1 out]
            n194 = call <vilib>:"Serial Port Read.vi"("requested byte count"=w691, "port number"=w683) -> ("string read"=w689:string)  [unwired: 1 out]
            n195 = Fract/Exp String To Number(string=w689) -> (number=w687:dbl)  [unwired: 3 in, 1 out]
            "atm" <- w687
            n196 = Multiply(x=w687, y=100.0) -> (x*y=w684:dbl)
            "%" <- w684
            n197 = Multiply(x=w684, y=7.6) -> (x*y=w686:dbl)
            "Torr" <- w686
          }
        }
        n198 = Wait (ms)(milliseconds to wait=w667) -> ()  [unwired: 1 out]
        n199 = Greater?(x=w670, y=1e-07) -> (0:w673:bool)
        n200 = case shown="False" w673 {
          tunnel: [w678 w679] -> w672
          tunnel: w670 -> [_ w679]
          tunnel: w671 -> [w678 _]
          frame False {
          }
          frame True {
          }
        }
        n201 = Number To Engineering String(4:w672) -> (0:w668:string)  [unwired: 3 in]
        n202 = Bundle(w668) -> (w675:cluster{string})  [unwired: 1 in]
        n203 = Fract/Exp String To Number(string=w675) -> (number=→"Waveform Chart":cluster{dbl})  [unwired: 3 in, 1 out]
      }
    }
    n204 = Wait (ms)(milliseconds to wait=w267) -> ()  [unwired: 1 out]
    n205 = case "SRS QCM" shown="True" w288 {
      selector: w288 -> [w645 w651]
      tunnel: w291 -> [w649 w657]
      tunnel: w290 -> [w648 w659]
      tunnel: [w650 w664] -> w289
      tunnel: [w650 w663] -> w285
      tunnel: [w647 w662] -> w282
      tunnel: [0.0 w652] -> w247
      tunnel: [w645 w651] -> w255
      frame False {
        w650 = ""
        n206 = Bundle(w645, "VISA out"=w649, "error out"=w648) -> (w647:T13)  [unwired: 1 in]
      }
      frame True {
        # "SRS QCM"
        n207 = call "Elapsed Time2"() -> ("Elapsed Time (s)"=w658:dbl)  [unwired: 12 in, 7 out]
        n208 = call "SrsQcm200FandR_MODIFIED.vi"("VISA in"=w657, "Reference time in"=w658, "error in (no error)"=w659) -> ("VISA out"=w655:refnum<visa-resource-name>, "Frequency out"=w652:dbl, "Resistance out"=w654:dbl, "error out"=w656:errorcluster)  [unwired: 6 in, 3 out]
        "Ohm" <- w654
        n209 = Number To Engineering String(4:w654) -> (0:w663:string)  [unwired: 3 in]
        n210 = Divide(x=w652, y=1000000.0) -> (x/y=w653:dbl)
        "MHz" <- w653
        n211 = Number To Engineering String(4:w652) -> (0:w664:string)  [unwired: 3 in]
        n212 = Bundle(w653, "Resistance out"=w654) -> (→"Waveform Chart 7":cluster{dbl, "Resistance out":dbl})  [unwired: 1 in]
        n213 = Bundle(w651, "VISA out"=w655, "error out"=w656) -> (w662:T13)  [unwired: 1 in]
      }
    }
    n214 = case "Keithley 2420" shown="True" w264 {
      selector: w264 -> [w633 w641]
      tunnel: w293 -> [w632 w636]
      tunnel: w292 -> [w631 w635]
      tunnel: [w630 w639] -> w283
      tunnel: ["" w638] -> w284
      frame False {
        n215 = Bundle(w633, "VISA resource name out"=w632, "error out"=w631) -> (w630:T6)  [unwired: 1 in]
      }
      frame True {
        # "Keithley 2420"
        n216 = call-poly "Read.vi"("VISA resource name"=w636, "error in (no error)"=w635) -> ("VISA resource name out"=w642:refnum<visa-resource-name>, "Resistance"=w637:sgl, "error out"=w640:errorcluster)  [unwired: 7 in, 4 out]
        n217 = Bundle("Resistance"=w637) -> (→"Keithley 2420 (Ohm)":cluster{"Resistance":sgl})  [unwired: 1 in]
        n218 = Number To Engineering String(4:w637) -> (0:w638:string)  [unwired: 3 in]
        n219 = Wait (ms)(milliseconds to wait=u32 20) -> ()  [unwired: 1 out]
        n220 = Bundle(w641, "VISA resource name out"=w642, "error out"=w640) -> (w639:T6)  [unwired: 1 in]
      }
    }
    n221 = case "Keithley 6430" shown="True" w257 {
      selector: w257 -> [w582 w592]
      tunnel: w260 -> [w581 w589]
      tunnel: w259 -> [w580 w588]
      tunnel: ["" w591] -> w219
      tunnel: [w579 w590] -> w258
      frame False {
        n222 = Bundle(w582, "VISA resource name out"=w581, "error out"=w580) -> (w579:T6)  [unwired: 1 in]
      }
      frame True {
        # "Keithley 6430"
        n223 = call-poly "Read.vi"("error in (no error)"=w588, "VISA resource name"=w589) -> ("error out"=w587:errorcluster, "Measurement"=w585:dbl, "VISA resource name out"=w586:refnum<visa-resource-name>)  [unwired: 1 in, 6 out]
        n224 = Number To Engineering String(4:w585) -> (0:w591:string)  [unwired: 3 in]
        n225 = Bundle("Measurement"=w585) -> (→"Keithley 6430 (Ohm)":cluster{"Measurement":dbl})  [unwired: 1 in]
        n226 = Wait (ms)(milliseconds to wait=u32 20) -> ()  [unwired: 1 out]
        n227 = Bundle(w592, "VISA resource name out"=w586, "error out"=w587) -> (w590:T6)  [unwired: 1 in]
      }
    }
    n228 = Unbundle(w273) -> (w272:bool, "VISA resource name out"=w271:refnum<visa-resource-name>, "error out"=w270:errorcluster)
    n229 = call "J-KEM_subVI.vi"("Address in"=w280, "J-KEM on?"=w277) -> ("String data out"=w278:string, "plot data out"=→"J-Kem Temp (C)":cluster{"Numeric Control":dbl}, "Address out"=w279:T14)  [unwired: 7 in]
    n230 = Greater?(x=w210, y=1.0) -> (0:w220:bool)
    n231 = case "RapidOX O2 Sensor" shown="True" w272 {
      tunnel: w271 -> [_ w603]
      tunnel: w270 -> [w596 w602]
      tunnel: ["" w601] -> w269
      tunnel: [w596 w598] -> w268
      frame False {
      }
      frame True {
        # "RapidOX 2100"
        n232 = VISA Write(VISA resource name=w603, write buffer="D", error in (no error)=w602) -> (VISA resource name out=w606:refnum<visa-resource-name>, error out=w605:errorcluster)  [unwired: 1 out]
        n233 = flat-sequence {
          tunnel: [w615] -> w612
          tunnel: [w613] -> w611
          tunnel: w606 -> [w615]
          tunnel: w605 -> [w613]
          tunnel: w612 -> [w620]
          tunnel: w611 -> [w619]
          tunnel: [w618] -> w610
          tunnel: [w617] -> w609
          tunnel: [w616] -> w608
          tunnel: w610 -> [w629]
          tunnel: w609 -> [w628]
          tunnel: w608 -> [w627]
          tunnel: [w626] -> w598
          tunnel: [w621] -> w600
          frame #0 {
            n234 = Wait (ms)(milliseconds to wait=u32 100) -> ()  [unwired: 1 out]
          }
          frame #1 {
            n235 = property class="Instr"(reference=w620, error in=w619) -> (reference out=w618:refnum<visa-resource-name>, error out=w616:errorcluster, "Bytes at Port"=w617:u32)
          }
          frame #2 {
            n236 = VISA Read(VISA resource name=w629, byte count=w628, error in (no error)=w627) -> (read buffer=w624:string, error out=w626:errorcluster)  [unwired: 2 out]
            n237 = Match Pattern(string=w624, regular expression="d") -> (after substring=w622:string)  [unwired: 1 in, 3 out]
            n238 = Match Pattern(string=w622, regular expression=",") -> (before substring=w621:string)  [unwired: 1 in, 3 out]
          }
        }
        n239 = flat-sequence {
          frame #0 {
          }
        }
        n240 = Fract/Exp String To Number(string=w600) -> (number=w599:dbl)  [unwired: 3 in, 1 out]
        "O2 Concentration (PPM)" <- w599
        n241 = Bundle(w599) -> (→"Waveform Chart 6":cluster{dbl})  [unwired: 1 in]
        n242 = Number To Engineering String(4:w599) -> (0:w601:string)  [unwired: 3 in]
      }
    }
    n243 = And(x=w220, y=w221) -> (x .and. y?=w232:bool)
    n244 = case shown="True" w232 {
      selector: w232 -> [w357 w388]
      tunnel: w231 -> [w359 w367]
      tunnel: w230 -> [w358 w368]
      tunnel: [w359 w371] -> w228
      tunnel: [w358 w370] -> w227
      tunnel: [w357 w388] -> w229
      tunnel: [w356 w369] -> w226
      tunnel: [w356 w362] -> w222
      tunnel: [w356 w366] -> w223
      frame False {
        w356 = ""
      }
      frame True {
        n245 = property class="Instr"(reference=w367, error in=w368) -> (reference out=w385:refnum<visa-resource-name>, error out=w387:errorcluster, "Bytes at Port"=w386:u32)
        n246 = VISA Read(VISA resource name=w385, byte count=w386, error in (no error)=w387) -> (VISA resource name out=w371:refnum<visa-resource-name>, read buffer=w360:string, error out=w370:errorcluster)  [unwired: 1 out]
        n247 = flat-sequence {
          tunnel: [w390] -> w361
          tunnel: w360 -> [w390]
          frame #0 {
            n248 = Wait (ms)(milliseconds to wait=u32 1500) -> ()  [unwired: 1 out]
          }
        }
        n249 = Search/Split String(string=w361, search string/char (-)=":") -> (match + rest of string=w382:string)  [unwired: 1 in, 2 out]
        n250 = Search/Split String(string=w382, offset (0)=1) -> (match + rest of string=w380:string)  [unwired: 1 in, 2 out]
        n251 = Search/Split String(string=w380, search string/char (-)="h") -> (substring before match=w369:string, match + rest of string=w378:string)  [unwired: 1 in, 1 out]
        "gas\nsensor" <- w369
        n252 = Search/Split String(string=w378, offset (0)=2) -> (match + rest of string=w376:string)  [unwired: 1 in, 2 out]
        n253 = Search/Split String(string=w376, search string/char (-)="t") -> (substring before match=w366:string, match + rest of string=w374:string)  [unwired: 1 in, 1 out]
        n254 = Search/Split String(string=w374, offset (0)=2) -> (match + rest of string=w364:string)  [unwired: 1 in, 2 out]
        n255 = Fract/Exp String To Number(string=w366) -> (number=w372:dbl)  [unwired: 3 in, 1 out]
        n256 = Bundle(w372) -> (→"Arduino humidity (%)":cluster{dbl})  [unwired: 1 in]
        n257 = Search/Split String(string=w364, search string/char (-)=".", offset (0)=0) -> (substring before match=w362:string)  [unwired: 2 out]
        "temp\n(C)" <- w362
      }
    }
    n258 = Select(t=w247, s=w249, f=w248) -> (s? t:f=w246:dbl)
    n259 = case shown="True" w255 {
      tunnel: w247 -> [_ w576]
      tunnel: ["" w574] -> w261
      tunnel: w246 -> [_ w573]
      frame False {
      }
      frame True {
        n260 = Subtract(x=w573, y=w576) -> (x-y=w577:dbl)
        n261 = Divide(x=w577, y=56.65) -> (x/y=w572:dbl)
        n262 = Bundle(w572) -> (→"QCM mass deposited (g)":cluster{dbl})  [unwired: 1 in]
        n263 = Number To Engineering String(4:w572) -> (0:w574:string)  [unwired: 3 in]
      }
    }
    n264 = Get Date/Time In Seconds() -> (seconds since 1Jan1904=w298:timestamp)
    n265 = Format Date/Time String(time format string (%c)="%Y-%m-%d %H:%M:%S%2u", seconds (now)=w298) -> (date/time string=w294:string)  [unwired: 1 in]
    n266 = Build Array(w294, w297, w219, w278, w284, w261, w289, w285, w286, w269, w245, w211, w244, w243, w226, w223, w222) -> (w225:string[])
  }
  n267 = Unbundle(w80) -> ("Boolean"=w79:bool, "VISA resource name out"=w78:refnum<visa-resource-name>, "error out"=w77:errorcluster)
  n268 = Unbundle(w85) -> (w84:bool, "VISA out"=w83:refnum<visa-resource-name>, "error out"=w82:errorcluster)
  n269 = Unbundle(w89) -> (w88:bool, "VISA resource name out"=w87:refnum<visa-resource-name>, "error out"=w86:errorcluster)
  n270 = case shown="True" w26 {
    tunnel: w25 -> [_ w693]
    tunnel: w24 -> [_ w694]
    frame False {
    }
    frame True {
      n271 = VISA Close(VISA resource name=w693, error in (no error)=w694) -> ()  [unwired: 1 out]
      n272 = call <vilib>:"Close.vi"("Arduino Resource"=T15 {"VISA resource"="", "Board Type"=enum."Uno", "Connection Type"=enum."USB / Serial", "Bytes Per Packet (15)"=15}) -> ()  [unwired: 14 in, 1 out]
    }
  }
  n273 = Unbundle(w51) -> (w56:bool, "VISA resource name out"=w55:refnum<visa-resource-name>, "error out"=w54:errorcluster)
  n274 = case shown="True" w43 {
    tunnel: [w695 w715] -> w41
    tunnel: w44 -> [_ w714]
    tunnel: w45 -> [_ w713]
    tunnel: w47 -> [_ w709]
    tunnel: w46 -> [_ w708]
    tunnel: [w695 w707] -> w42
    tunnel: [w696 w704] -> w40
    tunnel: w38 -> [w696 w703]
    tunnel: w30 -> [_ w700]
    tunnel: [w695 w699] -> w33
    tunnel: w32 -> [_ w698]
    tunnel: w31 -> [_ w697]
    frame False {
      w695 = errorcluster {"status"=FALSE, "code"=0, "source"=""} ("error out")
    }
    frame True {
      n275 = call <vilib>:"DAQmx Stop Task.vi"("task/channels in"=w698, "error in"=w697) -> ("task out"=w701:refnum<k21>, "error out"=w702:errorcluster)  [unwired: 12 in]
      n276 = call <vilib>:"DAQmx Stop Task.vi"("task/channels in"=w709, "error in"=w708) -> ("task out"=w711:refnum<k21>, "error out"=w710:errorcluster)  [unwired: 12 in]
      n277 = call <vilib>:"DAQmx Stop Task.vi"("task/channels in"=w714, "error in"=w713) -> ("task out"=w712:refnum<k21>, "error out"=w716:errorcluster)  [unwired: 12 in]
      n278 = VISA Clear(VISA resource name=w700, error in (no error)=w703) -> (VISA resource name out=w706:refnum<visa-resource-name>, error out=w705:errorcluster)
      n279 = call <vilib>:"DAQmx Clear Task.vi"("task in"=w701, "error in"=w702) -> ("error out"=w699:errorcluster)  [unwired: 13 in]
      n280 = call <vilib>:"DAQmx Clear Task.vi"("task in"=w711, "error in"=w710) -> ("error out"=w707:errorcluster)  [unwired: 13 in]
      n281 = call <vilib>:"DAQmx Clear Task.vi"("task in"=w712, "error in"=w716) -> ("error out"=w715:errorcluster)  [unwired: 13 in]
      n282 = VISA Close(VISA resource name=w706, error in (no error)=w705) -> (error out=w704:errorcluster)
    }
  }
  n283 = case shown="True" w88 {
    tunnel: w87 -> [_ w720]
    tunnel: w86 -> [w717 w719]
    tunnel: [w717 w718] -> w90
    frame False {
    }
    frame True {
      n284 = call "Enable Output.vi"("error in (no error)"=w719, "Enable Output (T: Enable)"=FALSE, "VISA resource name"=w720) -> ("error out"=w721:errorcluster, "VISA resource name out"=w723:refnum<visa-resource-name>)  [unwired: 7 in]
      n285 = call <vilib>:"Close.vi"("error in (no error)"=w721, "VISA resource name"=w723) -> ("error out"=w718:errorcluster)  [unwired: 9 in]
    }
  }
  n286 = case shown="True" w56 {
    tunnel: w55 -> [_ w726]
    tunnel: w54 -> [w724 w725]
    tunnel: [w724 w727] -> w50
    frame False {
    }
    frame True {
      w730 = FALSE  # Output (F:Off)
      n287 = call "Enable Output.vi"("error in (no error)"=w725, "Enable Output (F:Off)"=w730, "VISA resource name"=w726) -> ("error out"=w728:errorcluster, "VISA resource name out"=w729:refnum<visa-resource-name>)  [unwired: 7 out]
      n288 = call <vilib>:"Close.vi"("error in (no error)"=w728, "VISA resource name"=w729) -> ("error out"=w727:errorcluster)  [unwired: 9 out]
    }
  }
  n289 = case shown="False" w84 {
    tunnel: w82 -> [w731 w734]
    tunnel: [w731 w733] -> w91
    tunnel: w83 -> [_ w732]
    frame False {
    }
    frame True {
      n290 = call "srsQcm200Close.vi"("error in"=w734, "Visa in"=w732) -> ("error out"=w733:errorcluster)  [unwired: 3 in]
    }
  }
  n291 = case shown="True" w79 {
    tunnel: w78 -> [_ w738]
    tunnel: w77 -> [w735 w737]
    tunnel: [w735 w736] -> w76
    frame False {
    }
    frame True {
      n292 = VISA Close(VISA resource name=w738, error in (no error)=w737) -> (error out=w736:errorcluster)
    }
  }
  n293 = Merge Errors(w33, w42, w41, w40) -> (w39:errorcluster)
  n294 = Merge Errors(w50, w76, w90, w91, w61, w39) -> (w98:errorcluster)
  n295 = call <vilib>:"Simple Error Handler.vi"("error in (no error)"=w98) -> ()  [unwired: 4 in, 5 out]
  n296 = Build Array("date/time", "min elapsed", "Keithley 6430 resistance (Ohm)", "J-KEM temp (C)", "Keithley 2420 resistance (Ohm)" ("element"), "QCM adsorbed mass (g)", "QCM freq (Hz)", "QCM resistance (Ohm)", "O2 partial pressure (Torr)" ("element"), "O2 concentration (PPM)" ("element"), "chamber pressure (Torr)" ("element"), "chamber RH (%)" ("element"), "gas flow (sccm)" ("element"), "vapor flow (sccm)" ("element"), "gas sensor" ("element"), "humidity (%)" ("element"), "temp (C)" ("element"), "Experiment Notes") -> (w68:string[])
  n297 = call-poly <vilib>:"Write To Spreadsheet File.vi"("1D data"=w68, "file path (dialog if empty)"=w60) -> ("new file path (Not A Path if cancelled)"=w69:path)  [unwired: 6 in]
  n298 = call-poly <vilib>:"Write To Spreadsheet File.vi"("append to file? (new file:F)"=TRUE, "2D data"=w97, "file path (dialog if empty)"=w69) -> ()  [unwired: 5 in, 1 out]
